vi "DAQmx Create Channel (AI-Voltage-Custom with Excitation).vi"(0 "task in":refnum<k21>, 1 "maximum value":dbl=10.0 format="%0.2f", 2 "minimum value":dbl=-10.0 format="%0.2f", 3 "input terminal configuration":i32(ring)=-1 items=["default"=-1, "RSE"=10083, "NRSE"=10078, "Differential"=10106, "Pseudodifferential"=12529], 5 "physical channels":tag, 6 "use excitation for scaling":bool, 7 "name to assign":string, 9 "units":i32(ring)=10348 items=["Volts"=10348, "From Custom Scale"=10065], 10 "voltage excitation value":dbl format="%.6f", 11 "error in":errorcluster, 12 "custom scale name":tag, 13 "voltage excitation source":i32(ring)=10200 items=["Internal"=10200, "External"=10167, "None"=10230], 14 "bridge configuration":i32(ring)=10228 items=["Full Bridge"=10182, "Half Bridge"=10187, "Quarter Bridge"=10270, "No Bridge"=10228]) -> (4 "task out":refnum<k21>, 15 "error out":errorcluster)   [LabVIEW 2011]
doc: "Creates channel(s) to measure voltage. Use this instance for custom sensors that require excitation. You can use the excitation to scale the measurement."
uses:
  C:/Program Files/National Instruments/LabVIEW 2011/resource/objmgr/daqmx.rc
panel:
  # "input limits"
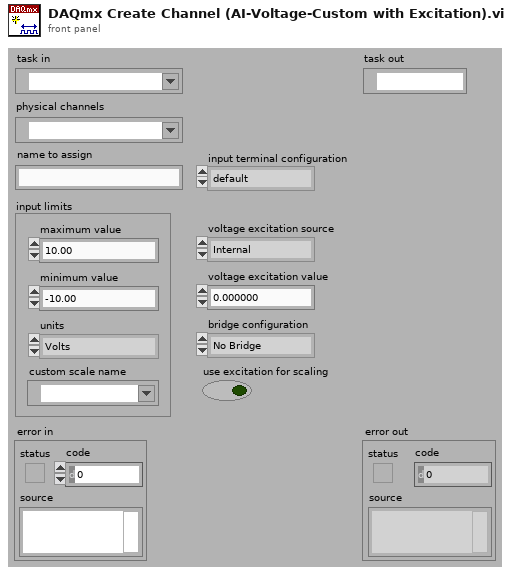
[diagram p1: front panel]
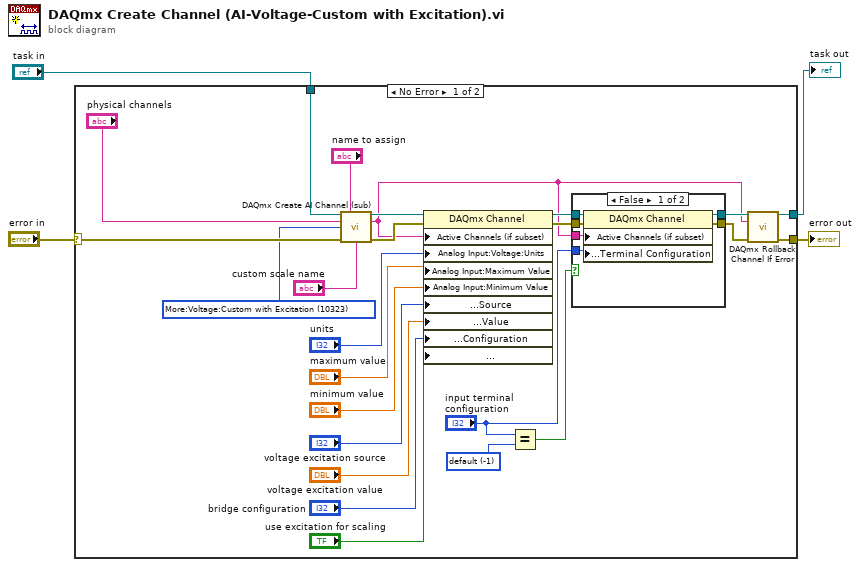
[diagram p0: block diagram]
diagram:
  n1 = case shown="No Error" "error in" {
    selector: "error in" -> [w28 w38]
    tunnel: [w7 w38] -> w4
    tunnel: "task in" -> [w29 w39]
    tunnel: [w6 w39] -> w1
    frame No Error {
      w14 = -1 items=["default"=-1, "differential"=10106, "RSE"=10083, "NRSE"=10078] ("input terminal configuration")
      w19 = 10323 items=["Voltage"=10322, "Current"=10134, "More:Voltage:Custom with Excitation"=10323, "More:Current:Custom with Excitation"=10136, "Frequency"=10181, "Period"=10257, "Resistance"=10278, "Temperature:Thermocouple"=10303, "Temperature:Thermistor"=10302, "Temperature:RTD"=10301, "Strain Gage"=10300] ("measurement type")
      n2 = call "DAQmx Create AI Channel (sub).vi"("task in"=w29, "virtual channel name"="name to assign", "physical channel name"="physical channels", "measurement type"=w19, "error in"=w28, "custom scale"="custom scale name") -> ("task out"=w12:refnum<k21>, "channel names"=w5:string, "error out"=w26:errorcluster)  [unwired: 7 out]
      n3 = property class="DAQmx Channel"(reference=w12, error in=w26, "Active Channels (if subset)"=w5, "Analog Input:Voltage:Units"="units", "Analog Input:Maximum Value"="maximum value", "Analog Input:Minimum Value"="minimum value", "Analog Input:General Properties:Signal Conditioning:Excitation:Source"="voltage excitation source", "Analog Input:General Properties:Signal Conditioning:Excitation:Value"="voltage excitation value", "Analog Input:General Properties:Signal Conditioning:Bridge:Configuration"="bridge configuration", "Analog Input:General Properties:Signal Conditioning:Excitation:Advanced:Use Excitation For Scaling"="use excitation for scaling") -> (reference out=w21:refnum<k21>, error out=w20:errorcluster)
      n4 = Equal?(x="input terminal configuration", y=w14) -> (x = y?=w22:bool)
      n5 = case shown="False" w22 {
        tunnel: "input terminal configuration" -> [w32 _]
        tunnel: w21 -> [w30 w37]
        tunnel: w20 -> [w35 w36]
        tunnel: [w34 w37] -> w9
        tunnel: [w33 w36] -> w8
        tunnel: w5 -> [w31 _]
        frame False {
          n6 = property class="DAQmx Channel"(reference=w30, error in=w35, "Active Channels (if subset)"=w31, "Analog Input:General Properties:Input Configuration:Terminal Configuration"=w32) -> (reference out=w34:refnum<k21>, error out=w33:errorcluster)
        }
        frame True {
        }
      }
      n7 = call "DAQmx Rollback Channel If Error.vi"("task in"=w9, "channel names"=w5, "error in"=w8) -> ("task out"=w6:refnum<k21>, "error out"=w7:errorcluster)  [unwired: 11 out]
    }
    frame Error {
    }
  }
  "error out" <- w4
  "task out" <- w1
